vi "Read_Gravi.vi"(0 "COM Bluegiga in":refnum<visa-resource-name>, 11 "error in (no error)":errorcluster) -> (4 "COM Bluegiga out":refnum<visa-resource-name>, 12 "X":sgl, 13 "Y":sgl, 14 "Z":ext, 15 "error out":errorcluster)   [LabVIEW 2020]
panel:
  out "(hi.lo)":u32
  out "characteristic value":u8[](array[numeric])
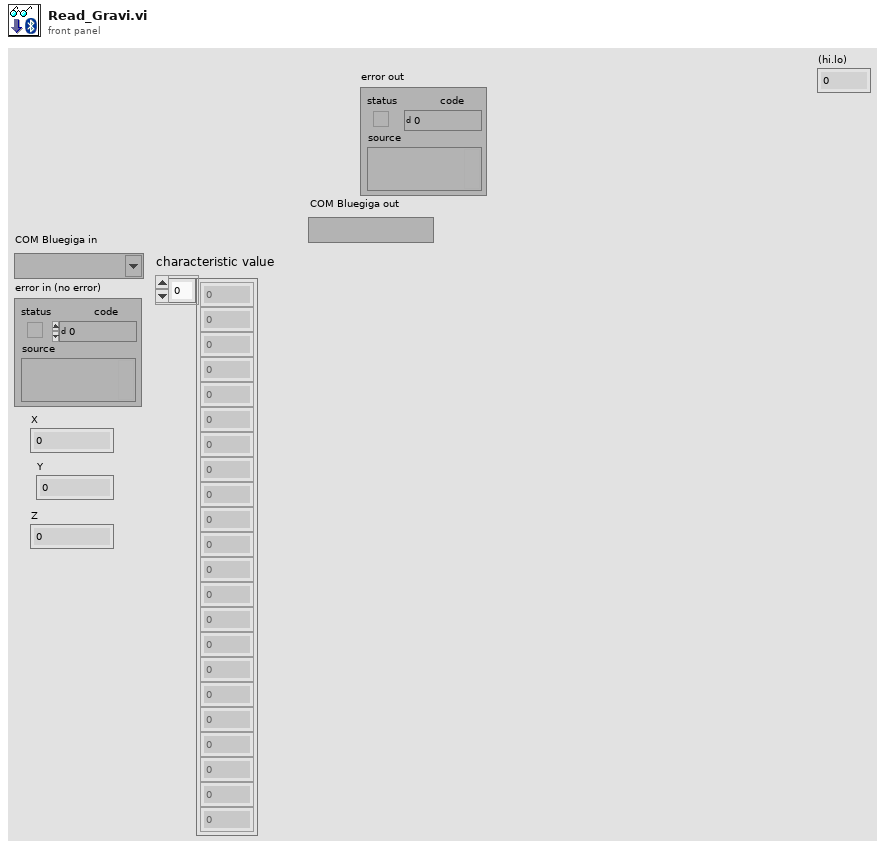
[diagram p1: front panel]
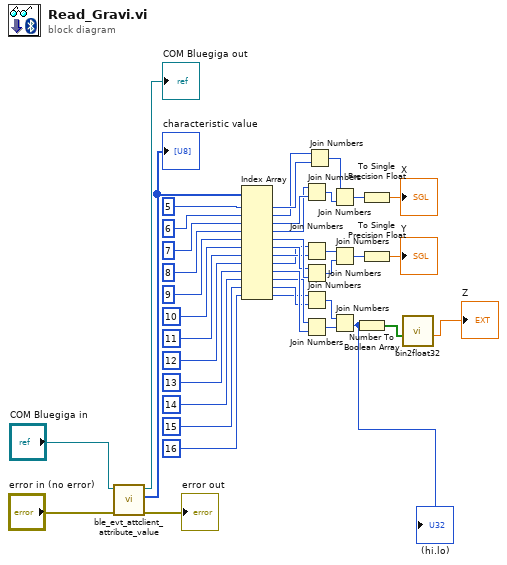
[diagram p0: block diagram]
diagram:
  n1 = call <vilib>:"ble_evt_attclient_attribute_value.vi"("error in (no error)"="error in (no error)", "COM Bluegiga in"="COM Bluegiga in") -> ("error out"=→"error out":errorcluster, "characteristic value"=w42:u8[], "COM Bluegiga out"=→"COM Bluegiga out":refnum<visa-resource-name>)  [unwired: 6 in, 1 out]
  "characteristic value" <- w42
  n2 = Index Array(array=w42, index #1=5 ("index"), index #2=6 ("index"), index #3=7 ("index"), index #4=8 ("index"), index #5=9 ("index"), index #6=10 ("index"), index #7=11 ("index"), index #8=12 ("index"), index #9=13 ("index"), index #10=14 ("index"), index #11=15 ("index"), index #12=16 ("index")) -> (element #1=w27:u8, element #2=w26:u8, element #3=w25:u8, element #4=w24:u8, element #5=w23:u8, element #6=w22:u8, element #7=w21:u8, element #8=w20:u8, element #9=w17:u8, element #10=w16:u8, element #11=w15:u8, element #12=w14:u8)
  n3 = Join Numbers(hi=w24, lo=w25) -> ((hi.lo)=w5:u16)
  n4 = Join Numbers(hi=w20, lo=w21) -> ((hi.lo)=w18:u16)
  n5 = Join Numbers(hi=w22, lo=w23) -> ((hi.lo)=w19:u16)
  n6 = Join Numbers(hi=w14, lo=w15) -> ((hi.lo)=w12:u16)
  n7 = Join Numbers(hi=w16, lo=w17) -> ((hi.lo)=w13:u16)
  n8 = Join Numbers(hi=w26, lo=w27) -> ((hi.lo)=w4:u16)
  n9 = Join Numbers(hi=w4, lo=w5) -> ((hi.lo)=w11:u32)
  n10 = Join Numbers(hi=w18, lo=w19) -> ((hi.lo)=w8:u32)
  n11 = Join Numbers(hi=w12, lo=w13) -> ((hi.lo)=w3:u32)
  "(hi.lo)" <- w3
  n12 = Number To Boolean Array(number=w3) -> (Boolean array=w2:bool[])
  n13 = To Single Precision Float(number=w11) -> (single precision float=→"X":sgl)
  n14 = To Single Precision Float(number=w8) -> (single precision float=→"Y":sgl)
  n15 = call "bin2float32.vi"("Binary"=w2) -> ("Result"=→"Z":ext)  [unwired: 10 in]
